vi "spi_read_id_send_data.vi"(5 "COM":bool, 6 "byVdCmdHeaderLen":u16, 7 "VISA name":refnum<visa-resource-name>, 8 "error in":errorcluster, 9 "I2C_VD_BUFFER_RW":u16, 10 "I2C_SLAVE_ID":u8, 11 "cmd_std_header_t":T2) -> (0 "error out":errorcluster, 3 "return":i32)   [LabVIEW 2016]
uses:
  Global variable.vi
panel:
  in  "usb_ctl_info_t":T1
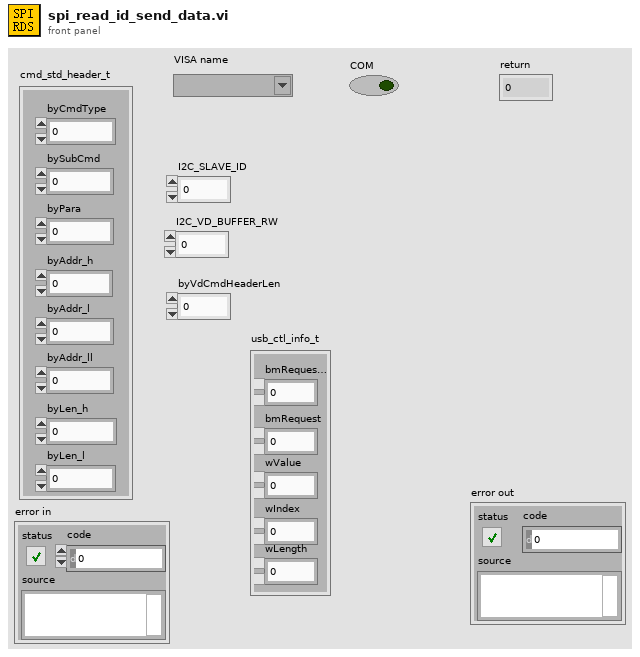
[diagram p1: front panel]
types:
  T1 = cluster{"bmRequestType":u8, "bmRequest":u8, "wValue":u16, "wIndex":u16, "wLength":u16}
  T2 = cluster{"byCmdType":u8, "bySubCmd":u8, "byPara":u8, "byAddr_h":u8, "byAddr_l":u8, "byAddr_ll":u8, "byLen_h":u8, "byLen_l":u8}
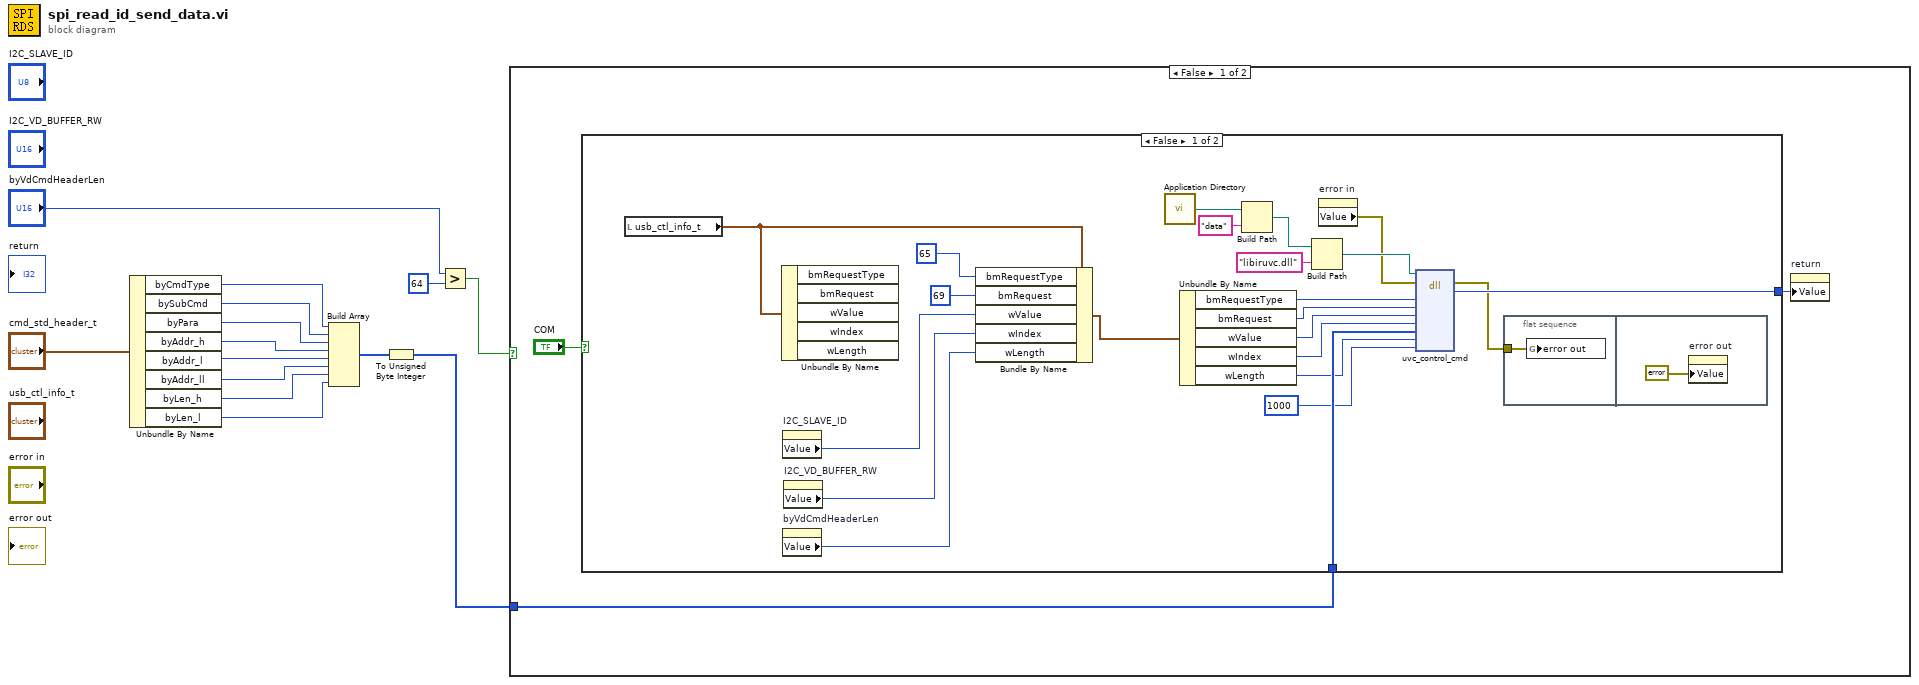
[diagram p0: block diagram]
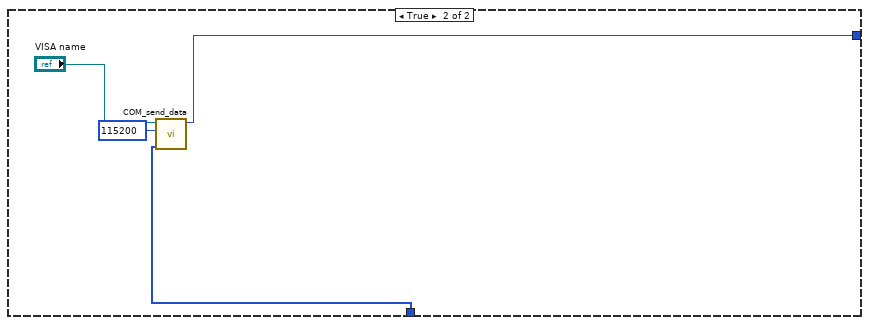
[diagram p2: hidden frame]
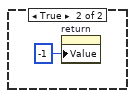
[diagram p3: hidden frame]
diagram:
  n1 = Unbundle By Name("cmd_std_header_t") -> ("byCmdType"=w13:u8, "bySubCmd"=w12:u8, "byPara"=w11:u8, "byAddr_h"=w10:u8, "byAddr_l"=w9:u8, "byAddr_ll"=w8:u8, "byLen_h"=w7:u8, "byLen_l"=w6:u8)
  n2 = Build Array(w13, w12, w11, w10, w9, w8, w7, w6) -> (w5:u8[])
  n3 = To Unsigned Byte Integer(number=w5) -> (unsigned 8bit integer=w1:u8[])
  n4 = Greater?(x="byVdCmdHeaderLen", y=u16 64) -> (0:w2:bool)
  n5 = case shown="False" w2 {
    tunnel: w1 -> [w17 _]
    frame False {
      n6 = case shown="False" "COM" {
        tunnel: w17 -> [w23 w45]
        tunnel: [w20 w42] -> w16
        frame False {
          n7 = local read "usb_ctl_info_t"() -> (w39:T1)
          n8 = Unbundle By Name(w39) -> ()  [unwired: 5 out]
          n9 = property on="I2C_SLAVE_ID" class="DigNum (strict)"() -> ("Value"=w36:u8)  [unwired: 2 in, 2 out]
          n10 = property on="byVdCmdHeaderLen" class="DigNum (strict)"() -> ("Value"=w34:u16)  [unwired: 2 in, 2 out]
          n11 = property on="I2C_VD_BUFFER_RW" class="DigNum (strict)"() -> ("Value"=w35:u16)  [unwired: 2 in, 2 out]
          n12 = Bundle By Name(cluster=w39, "bmRequestType"=u8 65, "bmRequest"=u8 69, "wValue"=w36, "wIndex"=w35, "wLength"=w34) -> (w28:T1)
          n13 = call <vilib>:"Application Directory.vi"() -> ("Application Directory"=w32:path)
          n14 = Unbundle By Name(w28) -> ("bmRequestType"=w27:u8, "bmRequest"=w26:u8, "wValue"=w25:u16, "wIndex"=w24:u16, "wLength"=w22:u16)
          n15 = Build Path(base path=w32, name or relative path="data") -> (appended path=w30:path)
          n16 = Build Path(base path=w30, name or relative path="libiruvc.dll") -> (appended path=w29:path)
          n17 = property on="error in" class="Clust (strict)"() -> ("Value"=w19:errorcluster)  [unwired: 2 in, 2 out]
          n18 = dll-call lib="PTH29abs EMyFolderISP上位机开发datalibiruvc.dll" fn="uvc_control_cmd"(path in=w29, error in=w19, "bmRequestType"=w27, "bRequest"=w26, "wValue"=w25, "wIndex"=w24, "data"=w23, "wLength"=w22, "timeout"=u32 1000) -> (error out=w18:errorcluster, "return type"=w20:i32)  [unwired: 8 in, 1 out]
          n19 = flat-sequence {
            tunnel: w18 -> [w40]
            frame #0 {
              n20 = global write "Global variable.vi" "error out"(w40) -> ()
            }
            frame #1 {
              n21 = property on="error out" class="Clust (strict)"("Value"=errorcluster {"status"=FALSE, "code"=0, "source"=""} ("error out")) -> ()  [unwired: 2 in, 2 out]
            }
          }
        }
        frame True {
          n22 = call "COM_send_data.vi"("data"=w45, "baud rate (9600)"=u32 115200, "VISA name"="VISA name") -> ("return"=w42:i32)  [unwired: 8 in]
        }
      }
      n23 = property on="return" class="DigNum (strict)"("Value"=w16) -> ()  [unwired: 2 in, 2 out]
    }
    frame True {
      n24 = property on="return" class="DigNum (strict)"("Value"=-1 ("return")) -> ()  [unwired: 2 in, 2 out]
    }
  }
